vi "Old Collector.vi"(0 "Clear":bool, 1 "FIRE":bool, 2 "REVERSE":bool, 3 "Intake Motor":bool, 4 "OVERRIDE":bool, 5 "OVERRIDE 2":bool, 8 "Intake":bool, 9 "1":bool, 10 "BB A/B":bool, 11 "2":bool, 12 "BB B":bool, 13 "3":bool, 14 "Prime":bool) -> (20 "Ball Count":dbl, 21 "Intake motor":dbl, 22 "Motor A":T1, 23 "Motor B":T1, 24 "Motor C":dbl)   [LabVIEW 2011]
uses:
  <vilib>/Rock Robotics/WPI/Relay/WPI_RelayValue.ctl
panel:
  in  "Fire Conveyor Speed to Fire":dbl(knob)=0.9023038992669639 scale=0.0..1.0
  in  "Intake Motor Speed":dbl(knob)=1.0 scale=0.0..1.0
  in  "Fire Conveyor Speed to Prime":dbl(knob)=0.21606338770259012 scale=0.0..1.0
  out "C from 3":bool
  out "B from 2":bool
  out "A from 1":bool
  out "BSB State":enum16{"Ball Entered"}(ring)
  out "BSC":bool
  out "BSB":bool
  out "BSA":bool
  out "MC":enum16{"Stopped", "Foward", "Reverse"}(ring)
  out "MA":enum16{"Stopped", "Foward", "Reverse"}(ring)
  out "MB":enum16{"Stopped", "Foward", "Reverse"}(ring)
  out "Intake motor":bool
  out "C Status":string
  out "B Status":string
  out "A Status":string
  out "Ball System State":string
  out "Primed":bool
  out "MA":bool
  out "MB":bool
  out "MC":bool
  # "Upper System"
  # "Upper/Middle System (U/M)"
  # "Ball systems"
  # "Vacant = Black (T)\nOccupied = Orange (F)"
  # "Lower/Middle System (L/M)"
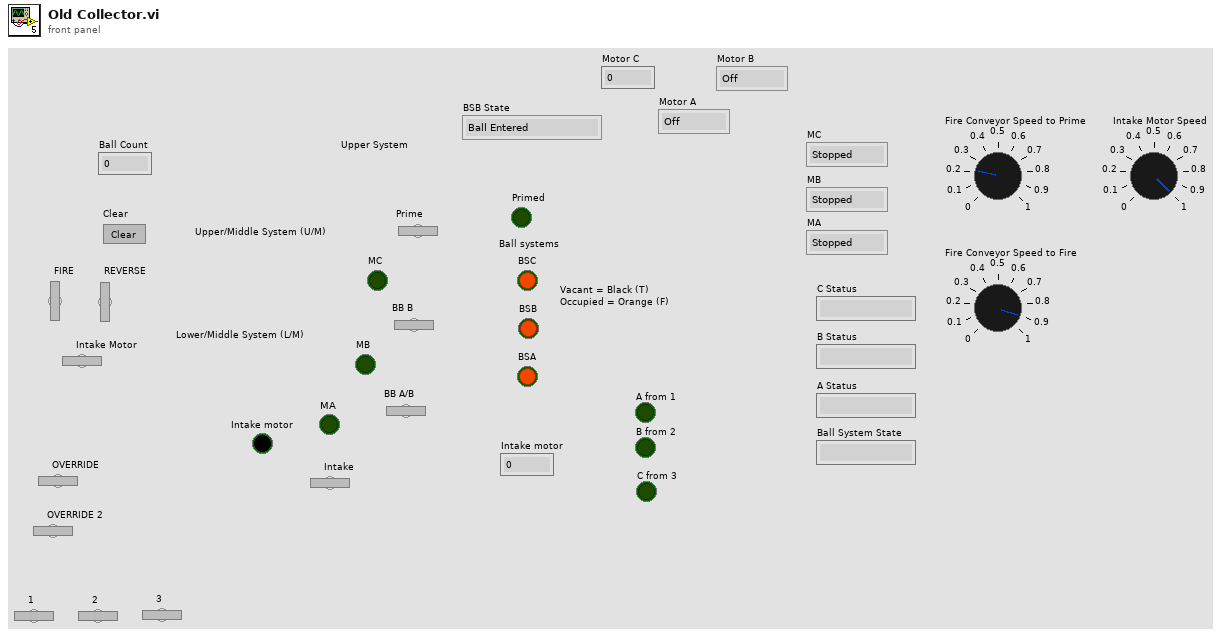
[diagram p1: front panel]
types:
  T1 = typedef "WPI_RelayValue.ctl" = enum16{"Off", "On", "Forward", "Reverse"}
  T2 = enum16{"Ball Entered", "Ball Stopped", "Ball Moveing", "Ball Leaving"}
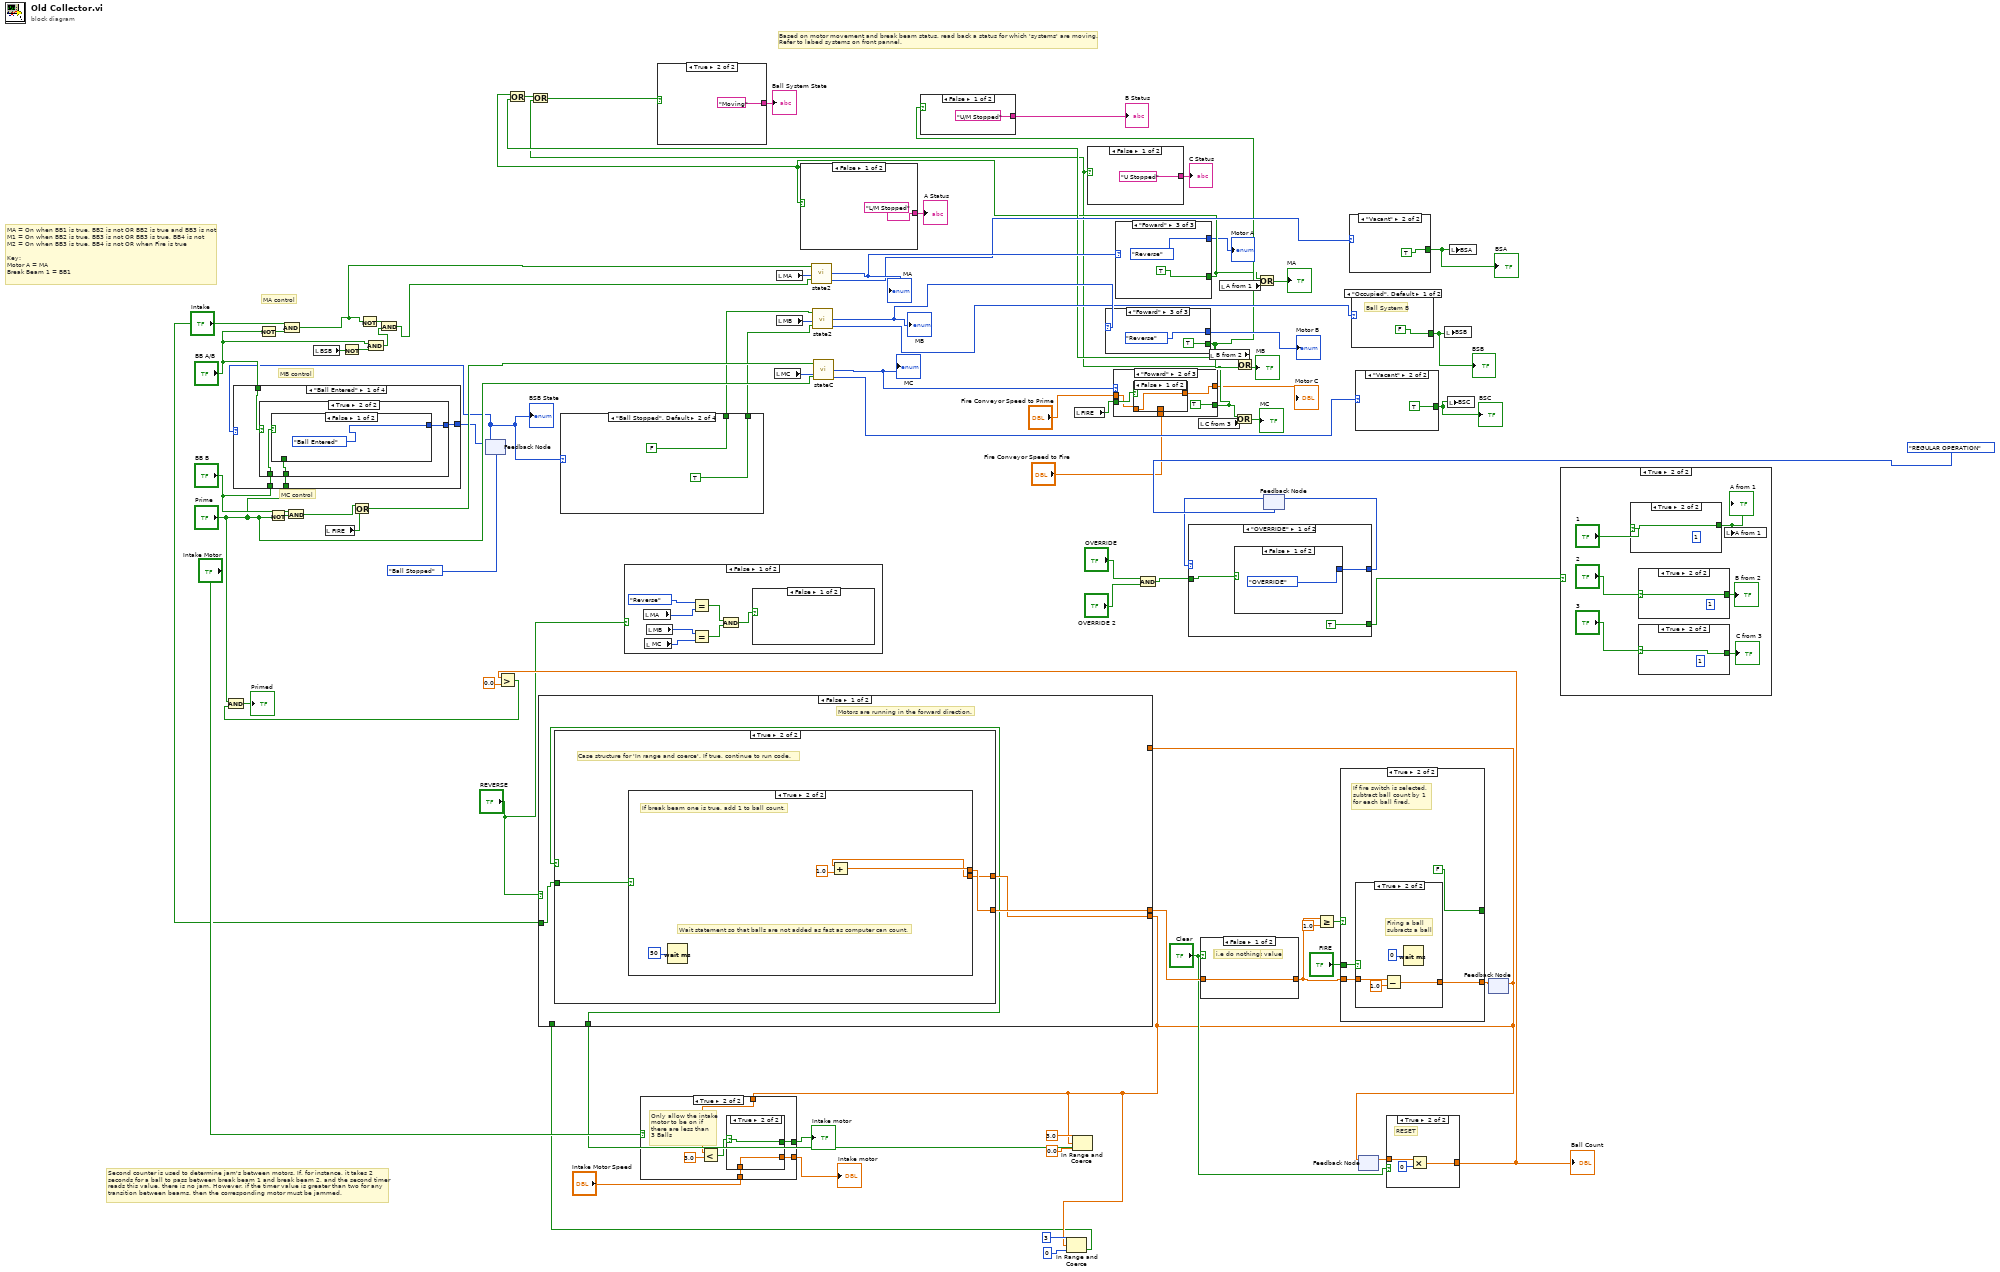
[diagram p0: block diagram]
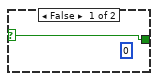
[diagram p3: hidden frame]
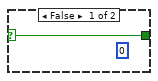
[diagram p4: hidden frame]
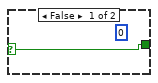
[diagram p5: hidden frame]
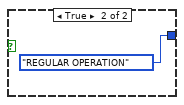
[diagram p6: hidden frame]
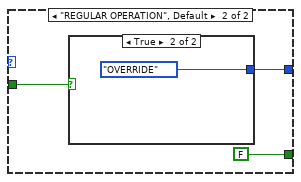
[diagram p7: hidden frame]
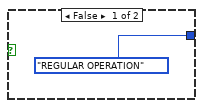
[diagram p8: hidden frame]
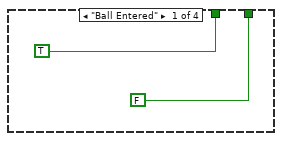
[diagram p9: hidden frame]
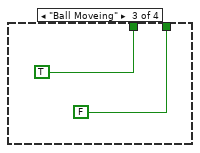
[diagram p10: hidden frame]
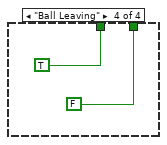
[diagram p11: hidden frame]
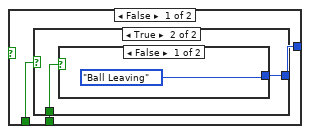
[diagram p12: hidden frame]
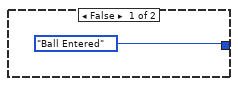
[diagram p13: hidden frame]
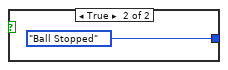
[diagram p14: hidden frame]
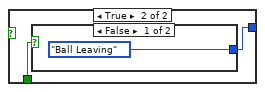
[diagram p15: hidden frame]
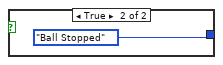
[diagram p16: hidden frame]
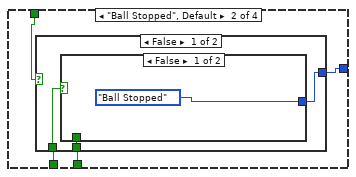
[diagram p17: hidden frame]
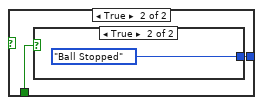
[diagram p18: hidden frame]
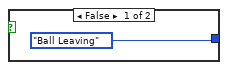
[diagram p19: hidden frame]
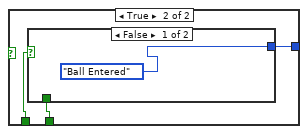
[diagram p20: hidden frame]
diagram:
  # "MC control"
  # "MB control"
  # "MA control"
  # "Second counter is used to determine jam's between motors. If, for instance, it takes 2\nseconds for a ball to pass between break beam 1 and break beam 2, and the second timer\nreads this value, there is no jam. However, if the timer value is greater than two for any\ntransition between beams, then the corresponding motor must be jammed."
  # "Based on motor movement and break beam status, read back a status for which 'systems' are moving.\nRefer to labed systems on front pannel."
  # "MA = On when BB1 is true, BB2 is not OR BB2 is true and BB3 is not\nM1 = On when BB2 is true, BB3 is not OR BB3 is true, BB4 is not\nM2 = On when BB3 is true, BB4 is not OR when Fire is true\n\nKey:\nMotor A = MA\nBreak Beam 1 = BB1"
  n1 = Not(x="BB A/B") -> (.not. x?=w52:bool)
  n2 = Not(x="Prime") -> (.not. x?=w51:bool)
  n3 = And(x="Intake", y=w52) -> (x .and. y?=w39:bool)
  n4 = And(x="BB B", y=w51) -> (x .and. y?=w50:bool)
  n5 = local read "BSB"() -> (w49:bool)
  n6 = local read "FIRE"() -> (w27:bool)
  n7 = Not(x=w49) -> (.not. x?=w48:bool)
  n8 = Or(x=w50, y=w27) -> (x .or. y?=w40:bool)
  n9 = Not(x=w39) -> (.not. x?=w45:bool)
  n10 = And(x="BB A/B", y=w48) -> (x .and. y?=w47:bool)
  n11 = And(x=w45, y=w47) -> (x .and. y?=w46:bool)
  n12 = feedback #1(T2."Ball Stopped") -> (w28:T2)
  "BSB State" <- w28
  n13 = case shown="\"Ball Entered\"" w28 {
    tunnel: "BB A/B" -> [w88 w108 w127 w145]
    tunnel: "BB B" -> [w87 w107 w126 w147]
    tunnel: "Prime" -> [w86 w106 w125 w146]
    tunnel: [w85 w105 w128 w148] -> w29
    frame "Ball Entered" {
      n14 = case shown="True" w88 {
        tunnel: [w91 w99] -> w85
        tunnel: w87 -> [w90 w97]
        tunnel: w86 -> [w89 w98]
        frame False {
          n15 = case shown="True" w90 {
            tunnel: [T2."Ball Entered" w94] -> w91
            tunnel: w89 -> [_ w93]
            frame False {
            }
            frame True {
              n16 = case shown="False" w93 {
                tunnel: [T2."Ball Leaving" T2."Ball Stopped"] -> w94
                frame False {
                }
                frame True {
                }
              }
            }
          }
        }
        frame True {
          n17 = case shown="False" w97 {
            tunnel: [T2."Ball Entered" w102] -> w99
            tunnel: w98 -> [_ w101]
            frame False {
            }
            frame True {
              n18 = case shown="False" w101 {
                tunnel: [T2."Ball Leaving" T2."Ball Stopped"] -> w102
                frame False {
                }
                frame True {
                }
              }
            }
          }
        }
      }
    }
    frame "Ball Stopped", Default {
      n19 = case shown="False" w108 {
        tunnel: [w111 w119] -> w105
        tunnel: w107 -> [w110 w117]
        tunnel: w106 -> [w109 w118]
        frame False {
          n20 = case shown="False" w110 {
            tunnel: [T2."Ball Stopped" w114] -> w111
            tunnel: w109 -> [_ w113]
            frame False {
            }
            frame True {
              n21 = case shown="True" w113 {
                tunnel: [T2."Ball Leaving" T2."Ball Stopped"] -> w114
                frame False {
                }
                frame True {
                }
              }
            }
          }
        }
        frame True {
          n22 = case shown="False" w117 {
            tunnel: [T2."Ball Entered" w122] -> w119
            tunnel: w118 -> [_ w121]
            frame False {
            }
            frame True {
              n23 = case shown="True" w121 {
                tunnel: [T2."Ball Leaving" T2."Ball Stopped"] -> w122
                frame False {
                }
                frame True {
                }
              }
            }
          }
        }
      }
    }
    frame "Ball Moveing" {
      n24 = case shown="True" w127 {
        tunnel: [w131 w139] -> w128
        tunnel: w126 -> [w130 w137]
        tunnel: w125 -> [w129 w138]
        frame False {
          n25 = case shown="False" w130 {
            tunnel: [T2."Ball Stopped" w134] -> w131
            tunnel: w129 -> [_ w133]
            frame False {
            }
            frame True {
              n26 = case shown="True" w133 {
                tunnel: [T2."Ball Leaving" T2."Ball Stopped"] -> w134
                frame False {
                }
                frame True {
                }
              }
            }
          }
        }
        frame True {
          n27 = case shown="False" w137 {
            tunnel: [T2."Ball Entered" w142] -> w139
            tunnel: w138 -> [_ w141]
            frame False {
            }
            frame True {
              n28 = case shown="False" w141 {
                tunnel: [T2."Ball Leaving" T2."Ball Stopped"] -> w142
                frame False {
                }
                frame True {
                }
              }
            }
          }
        }
      }
    }
    frame "Ball Leaving" {
      n29 = case shown="True" w145 {
        tunnel: [w151 w159] -> w148
        tunnel: w147 -> [w150 w157]
        tunnel: w146 -> [w149 w158]
        frame False {
          n30 = case shown="False" w150 {
            tunnel: [T2."Ball Stopped" w154] -> w151
            tunnel: w149 -> [_ w153]
            frame False {
            }
            frame True {
              n31 = case shown="True" w153 {
                tunnel: [T2."Ball Leaving" T2."Ball Stopped"] -> w154
                frame False {
                }
                frame True {
                }
              }
            }
          }
        }
        frame True {
          n32 = case shown="True" w157 {
            tunnel: [T2."Ball Entered" w162] -> w159
            tunnel: w158 -> [_ w161]
            frame False {
            }
            frame True {
              n33 = case shown="False" w161 {
                tunnel: [T2."Ball Leaving" T2."Ball Stopped"] -> w162
                frame False {
                }
                frame True {
                }
              }
            }
          }
        }
      }
    }
  }
  n34 = feedback-in #1(w29) -> ()
  n35 = case shown="\"Ball Stopped\", Default" w28 {
    tunnel: [TRUE FALSE TRUE TRUE] -> w31
    tunnel: [FALSE TRUE FALSE FALSE] -> w30
    frame "Ball Entered" {
    }
    frame "Ball Stopped", Default {
    }
    frame "Ball Moveing" {
    }
    frame "Ball Leaving" {
    }
  }
  n36 = case shown="False" "REVERSE" {
    frame False {
      n37 = local read "MA"() -> (w178:enum16{"Stopped", "Foward", "Reverse"})
      n38 = local read "MC"() -> (w176:enum16{"Stopped", "Foward", "Reverse"})
      n39 = local read "MB"() -> (w177:enum16{"Stopped", "Foward", "Reverse"})
      n40 = Equal?(x=enum16{"Stopped", "Foward", "Reverse"}."Reverse" ("value"), y=w178) -> (x = y?=w174:bool)
      n41 = Equal?(x=w177, y=w176) -> (x = y?=w175:bool)
      n42 = And(x=w174, y=w175) -> (x .and. y?=w173:bool)
      n43 = case shown="False" w173 {
        frame False {
        }
        frame True {
          w180 = enum16{"Stopped", "Foward", "Reverse"}."Stopped" ("value")
          n44 = local write "MA"(w180) -> ()
          n45 = local write "MB"(w180) -> ()
          n46 = local write "MC"(w180) -> ()
        }
      }
    }
    frame True {
      w181 = enum16{"Stopped", "Foward", "Reverse"}."Reverse" ("MB")
      n47 = local write "MC"(w181) -> ()
      n48 = local write "MA"(w181) -> ()
      n49 = local write "MB"(w181) -> ()
    }
  }
  n50 = local read "MC"() -> (w64:enum16{"Stopped", "Foward", "Reverse"})
  n51 = local read "MA"() -> (w65:enum16{"Stopped", "Foward", "Reverse"})
  n52 = local read "MB"() -> (w66:enum16{"Stopped", "Foward", "Reverse"})
  n53 = call "state2.vi"("Stop/Transfer"=w46, "State"=w65, "Start"=w39) -> ("Ball State"=w56:enum16{"Occupied", "Vacant"}, "OutState"=w63:enum16{"Stopped", "Foward", "Reverse"})  [unwired: 1 in]
  "MA" <- w63
  n54 = call "state2.vi"("Stop/Transfer"=w30, "State"=w66, "Start"=w31) -> ("Ball State"=w57:enum16{"Occupied", "Vacant"}, "OutState"=w62:enum16{"Stopped", "Foward", "Reverse"})  [unwired: 1 in]
  "MB" <- w62
  n55 = call "stateC.vi"("Stop/Transfer"="Prime", "State"=w64, "Start"=w40) -> ("Ball State"=w58:enum16{"Occupied", "Vacant"}, "OutState"=w60:enum16{"Stopped", "Foward", "Reverse"})  [unwired: 1 in]
  "MC" <- w60
  n56 = local read "FIRE"() -> (w2:bool)
  n57 = case shown="\"Foward\"" w62 {
    tunnel: [WPI_RelayValue."Off" ("RelayValue") WPI_RelayValue."Forward" ("RelayValue") WPI_RelayValue."Reverse" ("RelayValue")] -> w61
    tunnel: [FALSE TRUE TRUE] -> w38
    frame "Stopped", Default {
    }
    frame "Reverse" {
    }
    frame "Foward" {
    }
  }
  "Motor B" <- w61
  n58 = case shown="False" w38 {
    tunnel: ["U/M Stopped" "U/M Moving"] -> w77
    frame False {
    }
    frame True {
    }
  }
  "B Status" <- w77
  n59 = case shown="\"Foward\"" w60 {
    tunnel: [FALSE TRUE TRUE] -> w19
    tunnel: [0.0 w194 w199] -> w5
    tunnel: "Fire Conveyor Speed to Prime" -> [_ w192 w200]
    tunnel: w2 -> [_ w195 _]
    tunnel: "Fire Conveyor Speed to Fire" -> [_ w193 _]
    frame "Stopped", Default {
    }
    frame "Foward" {
      n60 = case shown="False" w195 {
        tunnel: [w197 w198] -> w194
        tunnel: w193 -> [_ w198]
        tunnel: w192 -> [w197 _]
        frame False {
        }
        frame True {
        }
      }
    }
    frame "Reverse" {
      n61 = Negate(x=w200) -> (-x=w199:dbl)
    }
  }
  "Motor C" <- w5
  n62 = case shown="False" w19 {
    tunnel: ["U Stopped" "Firing"] -> w76
    frame False {
    }
    frame True {
    }
  }
  "C Status" <- w76
  n63 = case shown="\"Foward\"" w63 {
    tunnel: [FALSE TRUE TRUE] -> w25
    tunnel: [WPI_RelayValue."Off" ("RelayValue") WPI_RelayValue."Forward" ("RelayValue") WPI_RelayValue."Reverse" ("RelayValue")] -> w6
    frame "Stopped", Default {
    }
    frame "Reverse" {
    }
    frame "Foward" {
    }
  }
  "Motor A" <- w6
  n64 = Or(x=w25, y=w38) -> (x .or. y?=w42:bool)
  n65 = Or(x=w42, y=w19) -> (x .or. y?=w41:bool)
  n66 = case shown="True" w41 {
    tunnel: ["Stopped" "Moving"] -> w79
    frame False {
    }
    frame True {
    }
  }
  "Ball System State" <- w79
  n67 = case shown="False" w25 {
    tunnel: ["L/M Stopped" "L/M Moving up"] -> w78
    frame False {
    }
    frame True {
    }
  }
  "A Status" <- w78
  n68 = And(x="OVERRIDE", y="OVERRIDE 2") -> (x .and. y?=w15:bool)
  n69 = local read "C from 3"() -> (w18:bool)
  n70 = local read "B from 2"() -> (w21:bool)
  n71 = local read "A from 1"() -> (w22:bool)
  n72 = Or(x=w19, y=w18) -> (x .or. y?=→"MC":bool)
  n73 = Or(x=w21, y=w38) -> (x .or. y?=→"MB":bool)
  n74 = Or(x=w25, y=w22) -> (x .or. y?=→"MA":bool)
  n75 = feedback #2(enum16{"OVERRIDE", "REGULAR OPERATION"}."REGULAR OPERATION") -> (w16:enum16{"OVERRIDE", "REGULAR OPERATION"})
  n76 = case shown="\"OVERRIDE\"" w16 {
    tunnel: [w215 w221] -> w17
    tunnel: w15 -> [w216 w220]
    tunnel: [TRUE FALSE] -> w14
    frame "OVERRIDE" {
      n77 = case shown="False" w216 {
        tunnel: [enum16{"OVERRIDE", "REGULAR OPERATION"}."OVERRIDE" enum16{"OVERRIDE", "REGULAR OPERATION"}."REGULAR OPERATION"] -> w215
        frame False {
        }
        frame True {
        }
      }
    }
    frame "REGULAR OPERATION", Default {
      n78 = case shown="True" w220 {
        tunnel: [enum16{"OVERRIDE", "REGULAR OPERATION"}."REGULAR OPERATION" enum16{"OVERRIDE", "REGULAR OPERATION"}."OVERRIDE"] -> w221
        frame False {
        }
        frame True {
        }
      }
    }
  }
  n79 = feedback-in #2(w17) -> ()
  n80 = case shown="\"Vacant\"" w56 {
    tunnel: [FALSE TRUE] -> w54
    frame "Occupied", Default {
      # "Ball System A"
    }
    frame "Vacant" {
    }
  }
  "BSA" <- w54
  n81 = case shown="\"Occupied\", Default" w57 {
    tunnel: [FALSE TRUE] -> w55
    frame "Occupied", Default {
      # "Ball System B"
    }
    frame "Vacant" {
    }
  }
  "BSB" <- w55
  n82 = case shown="\"Vacant\"" w58 {
    tunnel: [FALSE TRUE] -> w53
    frame "Occupied", Default {
      # "Ball System C"
    }
    frame "Vacant" {
    }
  }
  "BSC" <- w53
  n83 = feedback #3() -> (w72:dbl)  [unwired: 1 in]
  n84 = case shown="True" "Clear" {
    tunnel: w72 -> [w230 w233]
    tunnel: [w230 w231] -> w67
    frame False {
      # "Feed Previous\nValue Through"
    }
    frame True {
      # "RESET"
      n85 = Multiply(x=w233, y=0) -> (x*y=w231:dbl)
    }
  }
  "Ball Count" <- w67
  n86 = Greater?(x=w67, y=0.0 ("f")) -> (0:w70:bool)
  n87 = And(x="Prime", y=w70) -> (x .and. y?=→"Primed":bool)
  n88 = local write "BSB"(w55) -> ()
  n89 = local write "BSC"(w53) -> ()
  n90 = local write "BSA"(w54) -> ()
  n91 = feedback #4() -> (w8:dbl)  [unwired: 1 in]
  n92 = case shown="True" "Intake Motor" {
    tunnel: w8 -> [_ w242]
    tunnel: [FALSE w239] -> w75
    tunnel: [w235 w238] -> w43
    tunnel: "Intake Motor Speed" -> [w234 w237]
    frame False {
      # "Intake Motor is off"
      n93 = Negate(x=w234) -> (-x=w235:dbl)
    }
    frame True {
      # "Only allow the intake\nmotor to be on if\nthere are less than\n3 Balls"
      n94 = Less?(x=w242, y=3.0) -> (x < y?=w240:bool)
      n95 = case shown="True" w240 {
        selector: w240 -> [_ w247]
        tunnel: [TRUE w247] -> w239
        tunnel: [w244 w246] -> w238
        tunnel: w237 -> [w243 w246]
        frame False {
          n96 = Negate(x=w243) -> (-x=w244:dbl)
        }
        frame True {
        }
      }
    }
  }
  "Intake motor" <- w75
  "Intake motor" <- w43
  n97 = In Range and Coerce(upper limit=3, x=w8, lower limit=0) -> (In Range?=w7:bool)  [unwired: 1 out]
  n98 = In Range and Coerce(upper limit=3.0, x=w8, lower limit=0.0) -> (In Range?=w11:bool)  [unwired: 1 out]
  n99 = case shown="False" "REVERSE" {
    tunnel: [w251 w265] -> w83
    tunnel: "Intake" -> [w249 w262]
    tunnel: w8 -> [w250 w264]
    tunnel: w8 -> [_ w263]
    tunnel: w11 -> [w248 _]
    tunnel: w7 -> [_ w261]
    frame False {
      # "Motors are running in the forward direction."
      n100 = case shown="True" w248 {
        tunnel: [w252 w255] -> w251
        tunnel: w250 -> [w252 w254]
        tunnel: w249 -> [_ w253]
        frame False {
          # "If ball count is not in range, stop code and disontinue intake."
        }
        frame True {
          # "Case structure for 'In range and coerce'. If true, continue to run code."
          n101 = case shown="True" w253 {
            tunnel: [w256 w258] -> w255
            tunnel: w254 -> [w256 w257]
            frame False {
              # "If break beam 1is not true, return previous value."
            }
            frame True {
              # "Wait statement so that balls are not added as fast as computer can count."
              # "If break beam one is true, add 1 to ball count."
              n102 = Wait (ms)(milliseconds to wait=u32 50) -> ()  [unwired: 1 out]
              n103 = Add(x=w257, y=1.0) -> (x+y=w258:dbl)
            }
          }
        }
      }
    }
    frame True {
      # "RUN MOTORS IN REVERSE\nA true constant is given to all motors to eject all balls."
      n104 = case shown="True" w261 {
        tunnel: [w268 w276] -> w265
        tunnel: w262 -> [w266 w274]
        tunnel: w264 -> [w267 w275]
        tunnel: w263 -> [_ w277]
        frame False {
          # "Wait statement added so that balls will not subtract as quickly as possible."
          # "If not in range, continue to eject balls in an instance where more than three are avaliable. There will never be a 'negative' ball count."
          n105 = Wait (ms)(milliseconds to wait=u32 1000) -> ()  [unwired: 1 out]
          n106 = case shown="True" w266 {
            tunnel: [w270 w272] -> w268
            tunnel: w267 -> [w270 w271]
            frame False {
              # "If Break Beam 1 is not tripped, run previous value through."
            }
            frame True {
              # "If true, continue to subtract from the ball count."
              n107 = Subtract(x=w271, y=1.0) -> (x-y=w272:dbl)
            }
          }
        }
        frame True {
          # "If ball count is indeed in range, continue to run motors in reverse until count reads 0 which is included in the range."
          n108 = case shown="True" w274 {
            tunnel: [w278 w283] -> w276
            tunnel: w275 -> [w278 w282]
            tunnel: w277 -> [_ w281]
            frame False {
              # "Run value through if break beam 1 is not true."
            }
            frame True {
              # "As long as ball count does not equal zero, \ncontinue to subtract balls until ball count reaches zero, \nincluded in the range."
              n109 = Not Equal To 0?(x=w281) -> (x != 0?=w280:bool)
              n110 = case shown="True" w280 {
                tunnel: [w284 w286] -> w283
                tunnel: w282 -> [w284 w285]
                frame False {
                }
                frame True {
                  n111 = Subtract(x=w285, y=1.0) -> (x-y=w286:dbl)
                }
              }
              n112 = Wait (ms)(milliseconds to wait=10.0) -> ()  [unwired: 1 out]
            }
          }
        }
      }
    }
  }
  n113 = case shown="False" "Clear" {
    tunnel: w83 -> [w288 _]
    tunnel: [w288 0] -> w81
    frame False {
      # "i.e do nothing"
      # "return previous value"
    }
    frame True {
      # "RESET"
    }
  }
  n114 = Greater Or Equal?(x=w81, y=1.0) -> (x >= y?=w82:bool)
  n115 = case shown="True" w82 {
    tunnel: [w290 w300] -> w68
    tunnel: w81 -> [w290 w299]
    tunnel: "FIRE" -> [w292 w298]
    tunnel: [w291 FALSE] -> _
    frame False {
      # "If fire switch has not been activated\nsend the previous value through and \ndo not subtract any ballz."
      n116 = case shown="True" w292 {
        tunnel: w290 -> [_ w296]
        tunnel: [FALSE w294] -> w291
        frame False {
        }
        frame True {
          n117 = Equal?(x=w296, y=0.0) -> (x = y?=w294:bool)
        }
      }
    }
    frame True {
      # "If fire switch is selected, \nsubtract ball count by 1 \nfor each ball fired."
      n118 = case shown="True" w298 {
        tunnel: [w301 w304] -> w300
        tunnel: w299 -> [w301 w303]
        frame False {
          # "Send Through"
        }
        frame True {
          # "Firing a ball\nsubracts a ball"
          n119 = Subtract(x=w303, y=1.0) -> (x-y=w304:dbl)
          n120 = Wait (ms)(milliseconds to wait=u32 0) -> ()  [unwired: 1 out]
        }
      }
    }
  }
  n121 = feedback-in #3(w8) -> ()
  n122 = feedback-in #4(w68) -> ()
  n123 = case shown="True" w14 {
    frame False {
    }
    frame True {
      n124 = case shown="True" "1" {
        selector: "1" -> [w316 w317]
        tunnel: [w316 w317] -> w308
        frame False {
          (unwired) 0
        }
        frame True {
          (unwired) 1
        }
      }
      "A from 1" <- w308
      n125 = case shown="True" "2" {
        selector: "2" -> [w314 w315]
        tunnel: [w314 w315] -> w306
        frame False {
          (unwired) 0
        }
        frame True {
          (unwired) 1
        }
      }
      "B from 2" <- w306
      n126 = case shown="True" "3" {
        selector: "3" -> [w312 w313]
        tunnel: [w312 w313] -> w307
        frame False {
          (unwired) 0
        }
        frame True {
          (unwired) 1
        }
      }
      "C from 3" <- w307
      n127 = local write "A from 1"(w308) -> ()
    }
  }
